vi "GetProperties.vi"(8 "error in":errorcluster, 11 "IOName in":refnum<class "IOName.lvclass">) -> (0 "error out":errorcluster, 3 "IOName out":refnum<class "IOName.lvclass">)   [LabVIEW 2014, in "Raspberry Pi Compatible Compiler for LabVIEW.lvlib" / "IOName.lvclass"]
uses:
  IOName.lvclass
  IOName.lvclass/IOName.ctl
  Control/Control.lvclass
  Text/Text.lvclass
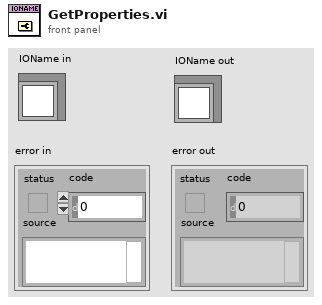
[diagram p1: front panel]
types:
  T1 = typedef "LVBoundsTypeDef.ctl" = cluster{"Width":u32, "Height":u32}
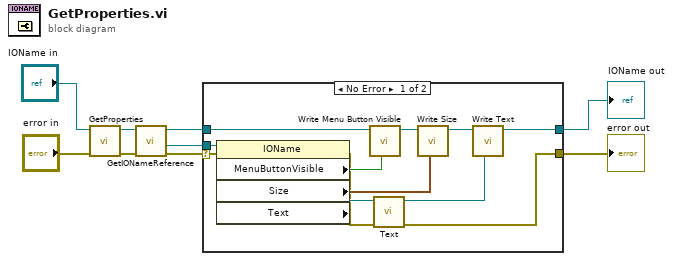
[diagram p0: block diagram]
diagram:
  n1 = call-parent "GetProperties.vi"("error in"="error in", "Control in"="IOName in") -> ("error out"=w6:errorcluster, "Control out"=w7:refnum<class "IOName.lvclass">)  [unwired: 8 in]
  n2 = call "GetIONameReference.vi"("error in"=w6, "IOName in"=w7) -> ("error out"=w5:errorcluster, "IOName reference"=w4:refnum<vi>, "IOName out"=w3:refnum<class "IOName.lvclass">)  [unwired: 7 in]
  n3 = case shown="No Error" w5 {
    selector: w5 -> [w21 w22]
    tunnel: w4 -> [w20 _]
    tunnel: w3 -> [w19 w23]
    tunnel: [w11 w23] -> w1
    tunnel: [w10 w22] -> w2
    frame No Error {
      n4 = property class="IOName"(reference=w20, error in=w21) -> (error out=w14:errorcluster, "MenuButtonVisible"=w18:bool, "Size"=w16:T1, "Text"=w15:refnum<vi>)  [unwired: 1 out]
      n5 = call "Write Menu Button Visible.vi"("Menu Button Visible"=w18, "IOName in"=w19) -> ("IOName out"=w17:refnum<class "IOName.lvclass">)  [unwired: 7 in]
      n6 = call "Text.vi"("error in"=w14, "Gen Refnum"=w15) -> ("error out"=w10:errorcluster, "Text out"=w12:refnum<class "Text.lvclass">)  [unwired: 8 in]
      n7 = call "Write Size.vi"("Size"=w16, "IOName in"=w17) -> ("IOName out"=w13:refnum<class "IOName.lvclass">)  [unwired: 7 in]
      n8 = call "Write Text.vi"("Text"=w12, "IOName in"=w13) -> ("IOName out"=w11:refnum<class "IOName.lvclass">)  [unwired: 7 in]
    }
    frame Error {
    }
  }
  "error out" <- w2
  "IOName out" <- w1
